vi "Add Cashier.vi"(7 "Time Scale [ms]":u32=3000, 8 "error in (no error)":errorcluster, 10 "Name":string, 11 "Coffee Shop in":refnum<class "Coffee Shop.lvclass">) -> (0 "error out":errorcluster, 3 "Coffee Shop out":refnum<class "Coffee Shop.lvclass">)   [LabVIEW 2020, in "Coffee Shop.lvclass"]
uses:
  Coffee Shop.lvclass
  People/Workers/Cashier/Cashier.lvclass
  C:/Git/astemes-triarc-examples/Coffee Shop/Processes/People/Person/Person.lvclass
  People/Person/Person.lvclass/Person.ctl
  <vilib>/Astemes/Triarc Framework/Process/Process.lvclass/Process.ctl
  <vilib>/Astemes/Triarc Framework/Process/Public/Lifecycle/Get Lifecycle State.vi
  <vilib>/Astemes/Triarc Framework/Process/Private/SubVIs/Handle Debug Data.vi
  <vilib>/Utility/error.llb/Clear Errors.vi
  <vilib>/Utility/High Resolution Relative Seconds.vi
  <vilib>/Utility/error.llb/Error Cluster From Error Code.vi
  Coffee Shop.lvclass/Coffee Shop.ctl
  People/Person/Person.lvclass
  C:/Git/astemes-triarc-examples/Coffee Shop/Processes/People/Workers/Worker/Worker.lvclass
  C:/Program Files (x86)/National Instruments/LabVIEW 2020/vi.lib/Astemes/Triarc Framework/View/View.lvclass
  C:/Program Files (x86)/National Instruments/LabVIEW 2020/vi.lib/Astemes/Triarc Framework/Process/Process.lvclass
  C:/Program Files (x86)/National Instruments/LabVIEW 2020/vi.lib/Astemes/Triarc Framework/Base/Base.lvclass
  C:/Program Files (x86)/National Instruments/LabVIEW 2020/vi.lib/Astemes/Triarc Framework/Error Handler Interface/Error Handler Interface.lvclass
  C:/Program Files (x86)/National Instruments/LabVIEW 2020/vi.lib/Astemes/Triarc Framework/Logging/Logging.lvclass
  C:/Git/astemes-triarc-examples/Coffee Shop/Processes/People/Process Job/Job Handler.lvclass
  C:/Git/astemes-triarc-examples/Coffee Shop/Processes/People/Workers/Cashier/Cashier.lvclass
  <vilib>/Astemes/Triarc Framework/Process/Process.lvclass
  C:/Program Files (x86)/National Instruments/LabVIEW 2020/vi.lib/Astemes/Triarc Framework/Application/Application.lvclass
  C:/Program Files (x86)/National Instruments/LabVIEW 2020/vi.lib/Astemes/Triarc Framework/Async Handler/Async Handler.lvclass
  C:/Git/astemes-triarc-examples/Coffee Shop/Processes/Coffee Shop/Coffee Shop.lvclass
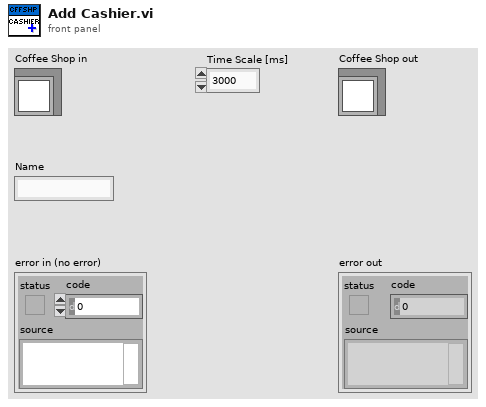
[diagram p1: front panel]
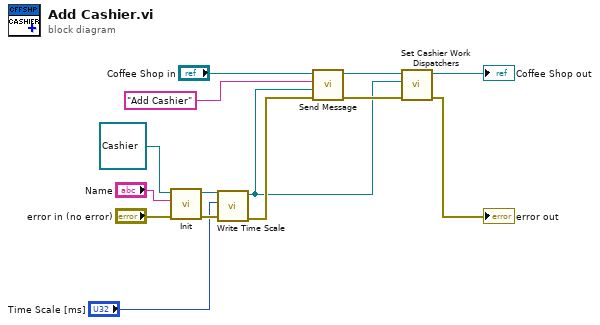
[diagram p0: block diagram]
diagram:
  n1 = call-dynamic "Init.vi"("error in (no error)"="error in (no error)", "Name"="Name", "View In"=refnum<class "Cashier.lvclass"> refnum ("Cashier.lvclass")) -> ("error out"=w8:errorcluster, "View Out"=w3:refnum<class "Cashier.lvclass">)  [unwired: 7 in]
  n2 = call "Write Time Scale.vi"("error in (no error)"=w8, "Time Scale [ms]"="Time Scale [ms]", "Person In"=w3) -> ("error out"=w4:errorcluster, "Person Out"=w2:refnum<class "Cashier.lvclass">)  [unwired: 7 in]
  n3 = call <vilib>:"Send Message.vi"("error in (no error)"=w4, "Message Data"=w2, "Message"="Add Cashier", "Process In"="Coffee Shop in") -> ("error out"=w14:errorcluster, "Process Out"=w6:refnum<class "Coffee Shop.lvclass">)  [unwired: 6 in]
  n4 = call "Set Cashier Work Dispatchers.vi"("error in (no error)"=w14, "Cashier"=w2, "Coffee Shop In"=w6) -> ("error out"=→"error out":errorcluster, "Coffee Shop Out"=→"Coffee Shop out":refnum<class "Coffee Shop.lvclass">)  [unwired: 7 in]
